vi "Generate Lithography Data.vi"(8 "error in (no error)":errorcluster, 11 "Tool Data in":refnum<class "Tool Data.lvclass">) -> (0 "error out":errorcluster, 2 "Lithography Data":T2(array[cluster]), 3 "Tool Data out":refnum<class "Tool Data.lvclass">)   [LabVIEW 2019, in "Tool Data.lvclass"]
uses:
  Tool Data.lvclass
  Tool Data.lvclass/Tool Data.ctl
  Tool Path/Tool Path.lvclass
  Settings/ObjectSettings/ObjectSettings.lvclass
  <userlib>/LevyLab/Relay Box/Typedefs/Resistor--enum.ctl
  <userlib>/LevyLab/Relay Box/Relay-Box.lvclass
  Tool Funnel/Tool Funnel.lvclass
  Tool Rectangle/Tool Rectangle.lvclass
  Tool Dot/Tool Dots.lvclass
  Settings/Path Settings/Path Settings.lvclass
  C:/Users/Albro/Documents/GitHub/AFM-Lithography/lvsrc/Classes/Settings/ObjectSettings/ObjectSettings.lvclass
  Settings/Funnel Settings/Funnel Settings.lvclass
  Settings/Rectangle Settings/Rectangle Settings.lvclass
  Settings/Dot Settings/Dot Settings.lvclass
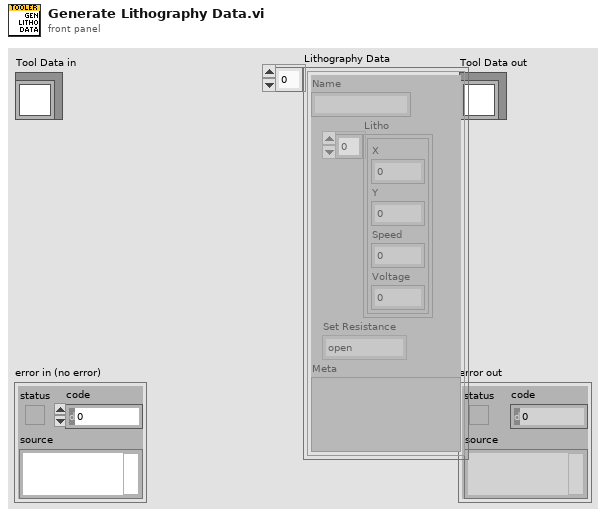
[diagram p1: front panel]
types:
  T1 = typedef "Relay-Box.lvclass/Resistor--enum.ctl" = enum16{"open", "discharge tip", "0 ohms", "100k ohm", "10M ohm", "1G ohm"}
  T2 = cluster{"Name":string, "Litho":cluster{"X":dbl, "Y":dbl, "Speed":dbl, "Voltage":dbl}[], "Set Resistance":T1, "Meta":variant}[]
  T3 = cluster{"Name":string, "Litho":cluster{"X":dbl, "Y":dbl, "Speed":dbl, "Voltage":dbl}[], "Set Resistance":T1, "Meta":variant}
  T4 = cluster{"X":dbl, "Y":dbl, "Speed":dbl, "Voltage":dbl}[]
  T5 = enum16{"Open", "Discharge Tip", "0 ohm", "100 kohm", "10 Mohm", "1 Gohm"}
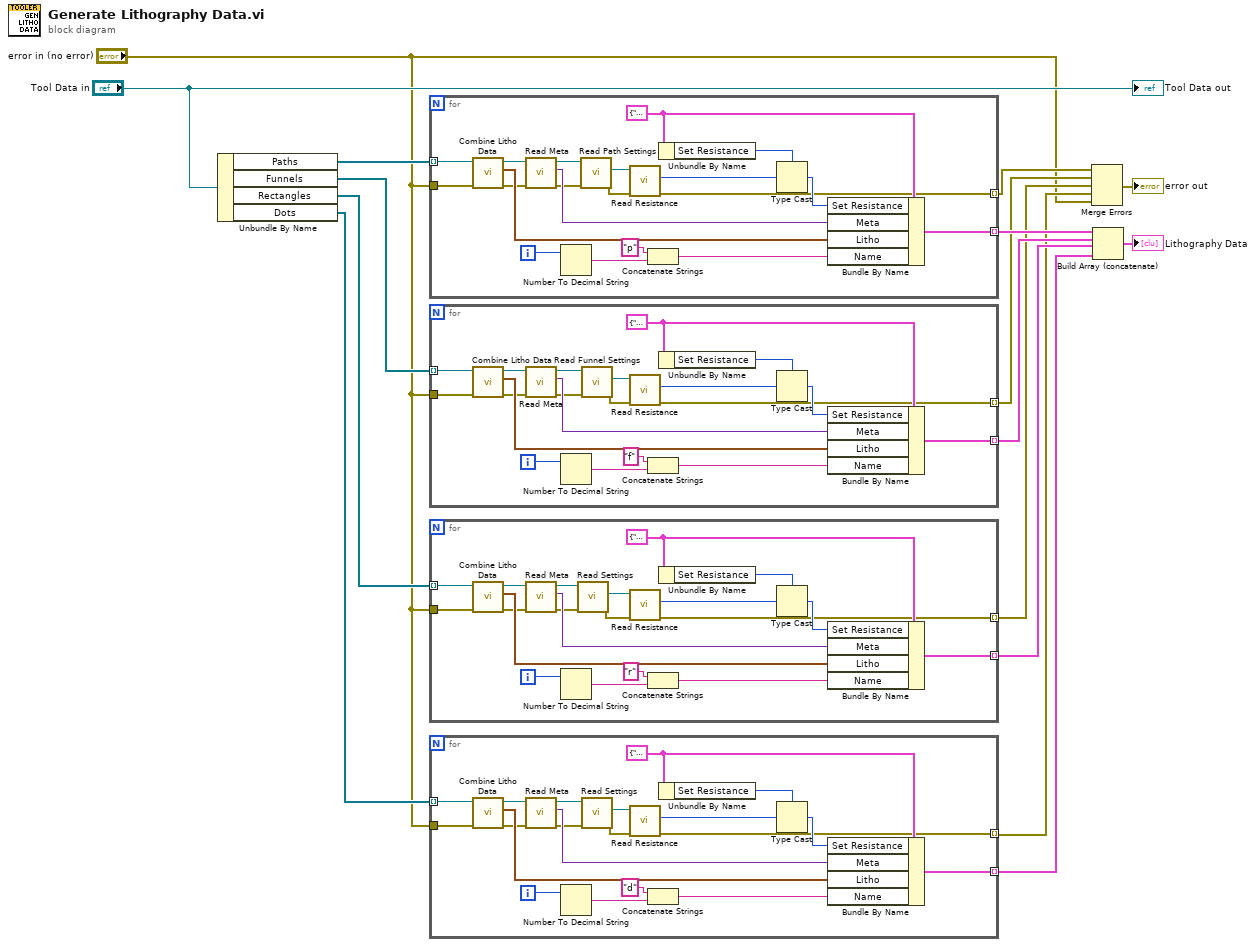
[diagram p0: block diagram]
diagram:
  n1 = Unbundle By Name("Tool Data in") -> ("Paths"=w15:refnum<class "Tool Path.lvclass">[], "Funnels"=w14:refnum<class "Tool Funnel.lvclass">[], "Rectangles"=w13:refnum<class "Tool Rectangle.lvclass">[], "Dots"=w12:refnum<class "Tool Dots.lvclass">[])
  n2 = for {
    tunnel: w15 -> [w36] mode=indexing
    tunnel: [w22] -> w11 mode=indexing
    tunnel: "error in (no error)" -> [w21]
    tunnel: [w20] -> w3 mode=indexing
    i -> [w31]
    w26 = T3 {"Name"="", "Litho"=[], "Set Resistance"=enum."1G ohm", "Meta"=variant} ("Pattern Data")
    n3 = call-dynamic "Combine Litho Data.vi"("error in (no error)"=w21, "Tool Object in"=w36) -> ("error out"=w19:errorcluster, "Output"=w29:T4, "Tool Object out"=w35:refnum<class "Tool Path.lvclass">)  [unwired: 7 in]
    n4 = call-dynamic "Read Meta.vi"("error in (no error)"=w19, "Tool Object in"=w35) -> ("error out"=w18:errorcluster, "Meta"=w28:variant, "Tool Object out"=w34:refnum<class "Tool Path.lvclass">)  [unwired: 7 in]
    n5 = Number To Decimal String(number=w31) -> (decimal integer string=w23:string)  [unwired: 1 in]
    n6 = call-dynamic "Read Path Settings.vi"("error in (no error)"=w18, "Tool Path in"=w34) -> ("error out"=w17:errorcluster, "Path Settings.lvclass"=w33:refnum<class "Path Settings.lvclass">)  [unwired: 7 in, 1 out]
    n7 = call "Read Resistance.vi"("error in (no error)"=w17, "ObjectSettings in"=w33) -> ("error out"=w20:errorcluster, "Resistance"=w27:T5)  [unwired: 7 in, 1 out]
    n8 = Concatenate Strings("p" ("string"), w23) -> (w30:string)
    n9 = Unbundle By Name(w26) -> ("Set Resistance"=w25:T1)
    n10 = Type Cast(type=w25, x=w27) -> (*(type *) &x=w24:T1)
    n11 = Bundle By Name(cluster=w26, "Set Resistance"=w24, "Meta"=w28, "Litho"=w29, "Name"=w30) -> (w22:T3)
  }
  n12 = for {
    tunnel: w14 -> [w56] mode=indexing
    tunnel: [w44] -> w10 mode=indexing
    tunnel: "error in (no error)" -> [w41]
    tunnel: [w40] -> w6 mode=indexing
    i -> [w53]
    w48 = T3 {"Name"="", "Litho"=[], "Set Resistance"=enum."1G ohm", "Meta"=variant} ("Pattern Data")
    n13 = call-dynamic "Combine Litho Data.vi"("error in (no error)"=w41, "Tool Object in"=w56) -> ("error out"=w39:errorcluster, "Output"=w51:T4, "Tool Object out"=w55:refnum<class "Tool Funnel.lvclass">)  [unwired: 7 in]
    n14 = call-dynamic "Read Meta.vi"("error in (no error)"=w39, "Tool Object in"=w55) -> ("error out"=w38:errorcluster, "Meta"=w50:variant, "Tool Object out"=w43:refnum<class "Tool Funnel.lvclass">)  [unwired: 7 in]
    n15 = Number To Decimal String(number=w53) -> (decimal integer string=w45:string)  [unwired: 1 in]
    n16 = call-dynamic "Read Funnel Settings.vi"("error in (no error)"=w38, "Tool Funnel in"=w43) -> ("error out"=w37:errorcluster, "Funnel Settings.lvclass"=w42:refnum<class "Funnel Settings.lvclass">)  [unwired: 7 in, 1 out]
    n17 = call "Read Resistance.vi"("error in (no error)"=w37, "ObjectSettings in"=w42) -> ("error out"=w40:errorcluster, "Resistance"=w49:T5)  [unwired: 7 in, 1 out]
    n18 = Concatenate Strings("f" ("string"), w45) -> (w52:string)
    n19 = Unbundle By Name(w48) -> ("Set Resistance"=w47:T1)
    n20 = Type Cast(type=w47, x=w49) -> (*(type *) &x=w46:T1)
    n21 = Bundle By Name(cluster=w48, "Set Resistance"=w46, "Meta"=w50, "Litho"=w51, "Name"=w52) -> (w44:T3)
  }
  n22 = for {
    tunnel: w13 -> [w76] mode=indexing
    tunnel: [w64] -> w9 mode=indexing
    tunnel: "error in (no error)" -> [w61]
    tunnel: [w60] -> w5 mode=indexing
    i -> [w73]
    w68 = T3 {"Name"="", "Litho"=[], "Set Resistance"=enum."1G ohm", "Meta"=variant} ("Pattern Data")
    n23 = call-dynamic "Combine Litho Data.vi"("error in (no error)"=w61, "Tool Object in"=w76) -> ("error out"=w59:errorcluster, "Output"=w71:T4, "Tool Object out"=w75:refnum<class "Tool Rectangle.lvclass">)  [unwired: 7 in]
    n24 = call-dynamic "Read Meta.vi"("error in (no error)"=w59, "Tool Object in"=w75) -> ("error out"=w58:errorcluster, "Meta"=w70:variant, "Tool Object out"=w63:refnum<class "Tool Rectangle.lvclass">)  [unwired: 7 in]
    n25 = Number To Decimal String(number=w73) -> (decimal integer string=w65:string)  [unwired: 1 in]
    n26 = call-dynamic "Read Settings.vi"("error in (no error)"=w58, "Tool Rectangle in"=w63) -> ("error out"=w57:errorcluster, "Rectangle Settings.lvclass"=w62:refnum<class "Rectangle Settings.lvclass">)  [unwired: 7 in, 1 out]
    n27 = call "Read Resistance.vi"("error in (no error)"=w57, "ObjectSettings in"=w62) -> ("error out"=w60:errorcluster, "Resistance"=w69:T5)  [unwired: 7 in, 1 out]
    n28 = Concatenate Strings("r" ("string"), w65) -> (w72:string)
    n29 = Unbundle By Name(w68) -> ("Set Resistance"=w67:T1)
    n30 = Type Cast(type=w67, x=w69) -> (*(type *) &x=w66:T1)
    n31 = Bundle By Name(cluster=w68, "Set Resistance"=w66, "Meta"=w70, "Litho"=w71, "Name"=w72) -> (w64:T3)
  }
  n32 = for {
    tunnel: w12 -> [w96] mode=indexing
    tunnel: [w84] -> w8 mode=indexing
    tunnel: "error in (no error)" -> [w81]
    tunnel: [w77] -> w4 mode=indexing
    i -> [w93]
    w88 = T3 {"Name"="", "Litho"=[], "Set Resistance"=enum."1G ohm", "Meta"=variant} ("Pattern Data")
    n33 = call-dynamic "Combine Litho Data.vi"("error in (no error)"=w81, "Tool Object in"=w96) -> ("error out"=w80:errorcluster, "Output"=w91:T4, "Tool Object out"=w95:refnum<class "Tool Dots.lvclass">)  [unwired: 7 in]
    n34 = call-dynamic "Read Meta.vi"("error in (no error)"=w80, "Tool Object in"=w95) -> ("error out"=w79:errorcluster, "Meta"=w90:variant, "Tool Object out"=w83:refnum<class "Tool Dots.lvclass">)  [unwired: 7 in]
    n35 = Number To Decimal String(number=w93) -> (decimal integer string=w85:string)  [unwired: 1 in]
    n36 = call-dynamic "Read Settings.vi"("error in (no error)"=w79, "Tool Dots in"=w83) -> ("error out"=w78:errorcluster, "Dot Settings.lvclass"=w82:refnum<class "Dot Settings.lvclass">)  [unwired: 7 in, 1 out]
    n37 = call "Read Resistance.vi"("error in (no error)"=w78, "ObjectSettings in"=w82) -> ("error out"=w77:errorcluster, "Resistance"=w89:T5)  [unwired: 7 in, 1 out]
    n38 = Concatenate Strings("d" ("string"), w85) -> (w92:string)
    n39 = Unbundle By Name(w88) -> ("Set Resistance"=w87:T1)
    n40 = Type Cast(type=w87, x=w89) -> (*(type *) &x=w86:T1)
    n41 = Bundle By Name(cluster=w88, "Set Resistance"=w86, "Meta"=w90, "Litho"=w91, "Name"=w92) -> (w84:T3)
  }
  n42 = Merge Errors(w3, w6, w5, w4, "error in (no error)") -> (→"error out":errorcluster)
  n43 = Build Array (concatenate)(w11, w10, w9, w8) -> (→"Lithography Data":T2)
  "Tool Data out" <- "Tool Data in"
